vi "stop.vi"(8 "error in (no error)":errorcluster, 11 "Display":refnum<class "DisplayBase.lvclass">) -> (0 "error out":errorcluster, 3 "CurrentConditionsDisplay.lvclass 2":refnum<class "DisplayBase.lvclass">)   [LabVIEW 2020, in "DisplayBase.lvclass"]
uses:
  DisplayBase.lvclass
  DisplayBase.lvclass/DisplayBase.ctl
panel:
  # "Connector Pane"
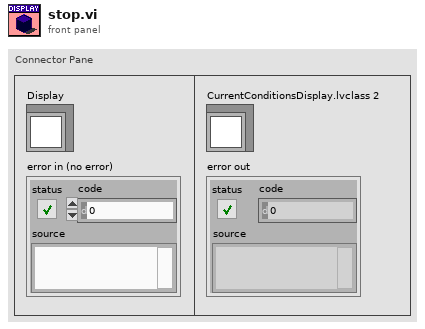
[diagram p1: front panel]
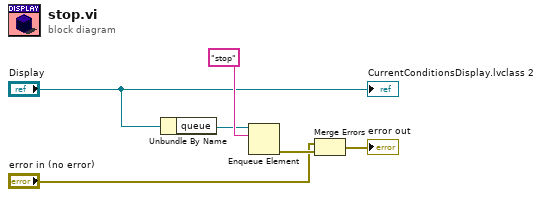
[diagram p0: block diagram]
diagram:
  n1 = Unbundle By Name("Display") -> ("queue"=w2:refnum<queue>)
  n2 = Enqueue Element(queue=w2, element="stop") -> (error out=w6:errorcluster)  [unwired: 2 in, 2 out]
  n3 = Merge Errors("error in (no error)", w6) -> (→"error out":errorcluster)
  "CurrentConditionsDisplay.lvclass 2" <- "Display"
